vi "MT8850 IVI Attribute.vi"(5 "Value (F)":bool, 7 "Set/Get (Set)":enum16{"Set", "Get"}(ring), 8 "error in (no error)":errorcluster, 10 "Flag (Simulate)":T1(ring), 11 "VISA session":refnum<visa-resource-name>) -> (0 "error out":errorcluster, 3 "VISA session out":refnum<visa-resource-name>, 4 "Value out":bool)   [LabVIEW 2017]
doc: "Whether the instrument is in single test or script mode."
uses:
  <instrlib>/aumt8852B/General/Utilities/Instrument.llb/Instrument Object Reference.ctl
panel:
  in  "reference":T2
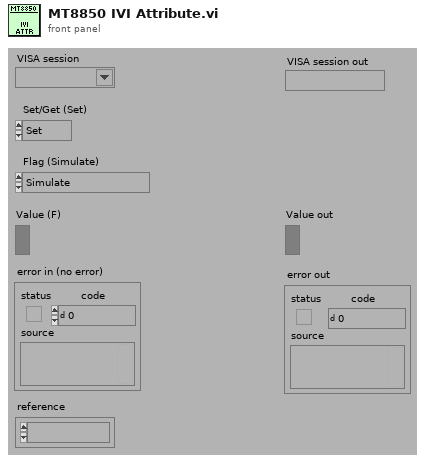
[diagram p1: front panel]
types:
  T1 = enum16{"Simulate", "Range check", "Cache", "Query instrument status"}
  T2 = typedef "Instrument Object Reference.ctl" = refnum<k1>
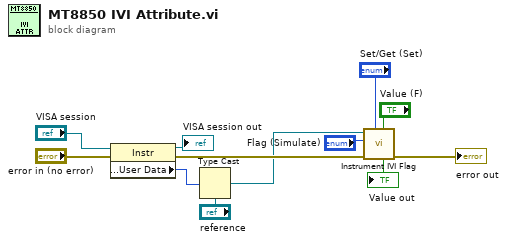
[diagram p0: block diagram]
diagram:
  n1 = property class="Instr"(reference="VISA session", error in="error in (no error)") -> (reference out=→"VISA session out":refnum<visa-resource-name>, error out=w9:errorcluster, "General Settings:User Data"=w8:u32)
  n2 = Type Cast(type="reference", x=w8) -> (*(type *) &x=w7:T2)
  n3 = call <instrlib>:"Instrument IVI Flag.vi"("Value (F)"="Value (F)", "Set/Get (Set)"="Set/Get (Set)", "error in (no error)"=w9, "Flag (Simulate)"="Flag (Simulate)", "reference"=w7) -> ("error out"=→"error out":errorcluster, "Value out"=→"Value out":bool)  [unwired: 4 in, 1 out]
